vi "ARI Control.vi"(4 "Joystick Values":T2) -> (1 "Lifter Status":T1)   [LabVIEW 2014]
uses:
  <vilib>/Rock Robotics/WPI/Relay/WPI_RelayValue.ctl
panel:
  in  "Lifter Status Def":T1
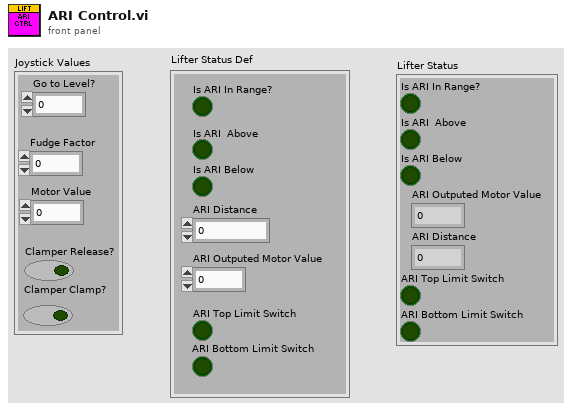
[diagram p1: front panel]
types:
  T1 = cluster{"Is ARI In Range?":bool, "Is ARI  Above":bool, "Is ARI Below":bool, "ARI Outputed Motor Value":dbl, "ARI Distance":dbl, "ARI Top Limit Switch":bool, "ARI Bottom Limit Switch":bool}
  T2 = cluster{"Go to Level?":i32, "Fudge Factor":dbl, "Clamper Release?":bool, "Motor Value":dbl, "Clamper Clamp?":bool}
  T3 = typedef "WPI_SwitchDevRef.ctl" = cluster{"DevStatus":errorcluster, "DIO Channel":T4, "Controller":T5, "CntIndex":T6, "Normally Closed":bool}
  T4 = typedef "FPGA_DIOChannel.ctl" = enum8{"DIO 0", "DIO 1", "DIO 2", "DIO 3", "DIO 4", "DIO 5", "DIO 6", "DIO 7", "DIO 8", "DIO 9", "DIO MXP 0", "DIO MXP 1", "DIO MXP 2", "DIO MXP 3", "DIO MXP 4", "DIO MXP 5", "DIO MXP 6", "DIO MXP 7", "DIO MXP 8", "DIO MXP 9", "DIO MXP 10", "DIO MXP 11", "DIO MXP 12", "DIO MXP 13", "DIO MXP 14", "DIO MXP 15", "Invalid"}
  T5 = typedef "FPGA_TypedefDigitalModule.ctl" = enum16{"Controller 1"}
  T6 = typedef "FPGA_CounterCtrSystemIndex.ctl" = enum8{"Ctr 0", "Ctr 1", "Ctr 2", "Ctr 3", "Ctr 4", "Ctr 5", "Ctr 6", "Ctr 7", "Invalid"}
  T7 = typedef "WPI_RelayValue.ctl" = enum16{"Off", "On", "Forward", "Reverse"}
  T8 = typedef "WPI_RelayDevRef.ctl" = cluster{"DevStatus":errorcluster, "Relay Channel":T9, "Controller":T5, "Relay Direction":T10}
  T9 = typedef "FPGA_DIORelayChannel.ctl" = enum8{"Relay 0", "Relay 1", "Relay 2", "Relay 3", "Invalid"}
  T10 = typedef "WPI_RelayDirection.ctl" = enum16{"Both directions", "Forward only", "Reverse only"}
  T11 = typedef "WPI_MotorControlDeviceRef.ctl" = cluster{"DeviceStatus":errorcluster, "Type":T12, "PWM":cluster{"Controller":T5, "PWM Channel":T13, "DeadBand":T14}, "CAN":cluster{"Device Number":u8, "Control Mode":T15, "Semaphore":T16, "Max Vout":dbl, "TalonSRX Control Mode":T17}, "Invert":bool, "TransformRef":T18, "InvTransformRef":T18}
  T12 = typedef "WPI_MotorControlType.ctl" = enum16{"PWM", "CAN", "CANTalonSRX"}
  T13 = typedef "FPGA_DIOPWMChannel.ctl" = enum8{"PWM 0", "PWM 1", "PWM 2", "PWM 3", "PWM 4", "PWM 5", "PWM 6", "PWM 7", "PWM 8", "PWM 9", "PWM MXP 0", "PWM MXP 1", "PWM MXP 2", "PWM MXP 3", "PWM MXP 4", "PWM MXP 5", "PWM MXP 6", "PWM MXP 7", "PWM MXP 8", "PWM MXP 9", "Invalid"}
  T14 = typedef "WPI_PWMDeadband.ctl" = cluster{"Name":string, "maxPositivePwm":i32, "minPositivePwm":i32, "centerPwm":i32, "maxNegativePwm":i32, "minNegativePwm":i32, "angularRange":u16}
  T15 = typedef "WPI_CANJaguar_ControlMode.ctl" = enum8{"Percent VBus", "Current", "Speed", "Position", "Voltage"}
  T16 = typedef "Semaphore RefNum" = refnum<k1>
  T17 = typedef "WPI_CANTalonSRX_APIControlMode.ctl" = enum8{"Percent VBus", "Speed", "Position", "Slave", "Unchanged / Invalid"}
  T18 = typedef "WPI_PWMTransform_ConPane.ctl" = refnum<vi>
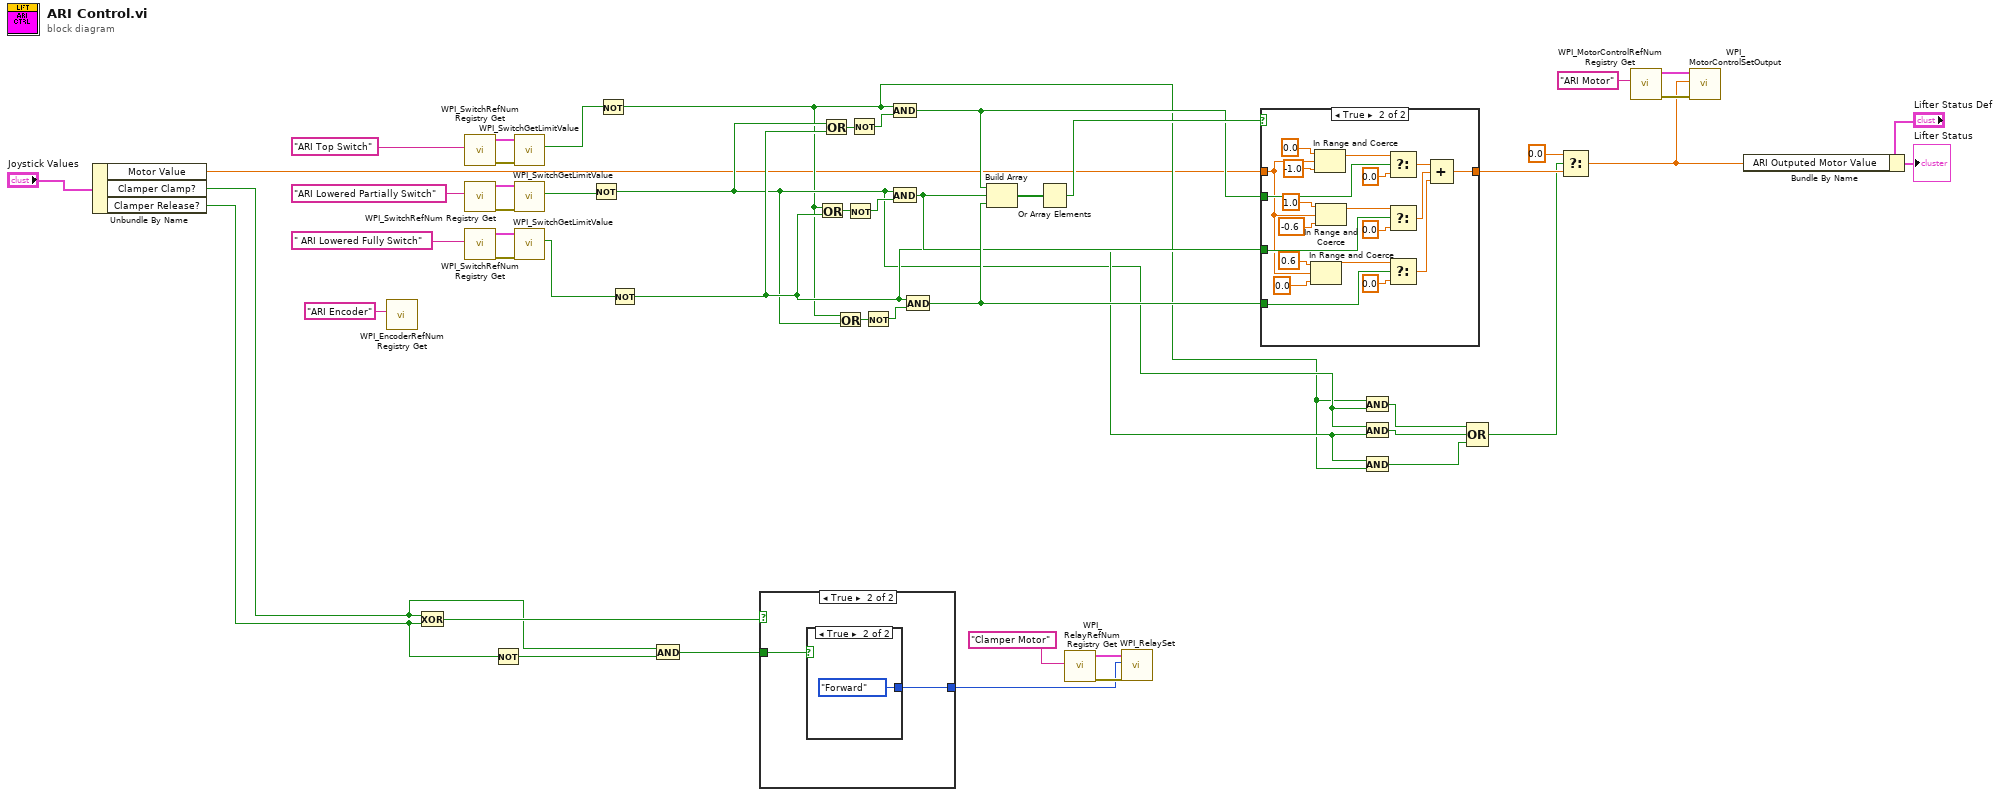
[diagram p0: block diagram]
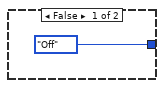
[diagram p3: hidden frame]
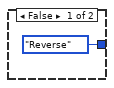
[diagram p4: hidden frame]
diagram:
  n1 = Unbundle By Name("Joystick Values") -> ("Motor Value"=w12:dbl, "Clamper Clamp?"=w2:bool, "Clamper Release?"=w4:bool)
  n2 = call <vilib>:"WPI_EncoderRefNum Registry Get.vi"("refnum name"="ARI Encoder") -> ()  [unwired: 9 in, 2 out]
  n3 = Exclusive Or(1:w4, 2:w2) -> (0:w6:bool)
  n4 = call <vilib>:"WPI_SwitchRefNum Registry Get.vi"("refnum name"="ARI Top Switch") -> ("error out"=w45:errorcluster, "SwitchDevRef"=w44:T3)  [unwired: 9 in]
  n5 = call <vilib>:"WPI_SwitchRefNum Registry Get.vi"("refnum name"="ARI Lowered Partially Switch") -> ("error out"=w42:errorcluster, "SwitchDevRef"=w43:T3)  [unwired: 9 in]
  n6 = call <vilib>:"WPI_SwitchRefNum Registry Get.vi"("refnum name"=" ARI Lowered Fully Switch") -> ("error out"=w38:errorcluster, "SwitchDevRef"=w37:T3)  [unwired: 9 in]
  n7 = Not(x=w4) -> (.not. x?=w3:bool)
  n8 = call <vilib>:"WPI_SwitchGetLimitValue.vi"("error in (no error)"=w45, "SwitchDevRef"=w44) -> ("Switch Pressed"=w9:bool)  [unwired: 7 in, 2 out]
  n9 = call <vilib>:"WPI_SwitchGetLimitValue.vi"("error in (no error)"=w42, "SwitchDevRef"=w43) -> ("Switch Pressed"=w10:bool)  [unwired: 7 in, 2 out]
  n10 = call <vilib>:"WPI_SwitchGetLimitValue.vi"("error in (no error)"=w38, "SwitchDevRef"=w37) -> ("Switch Pressed"=w11:bool)  [unwired: 7 in, 2 out]
  n11 = Not(x=w10) -> (.not. x?=w15:bool)
  n12 = Not(x=w9) -> (.not. x?=w14:bool)
  n13 = Not(x=w11) -> (.not. x?=w16:bool)
  n14 = And(x=w2, y=w3) -> (x .and. y?=w1:bool)
  n15 = case shown="True" w6 {
    tunnel: [WPI_RelayValue."Off" ("RelayValue") w52] -> w5
    tunnel: w1 -> [_ w53]
    frame False {
    }
    frame True {
      n16 = case shown="True" w53 {
        tunnel: [WPI_RelayValue."Reverse" ("RelayValue") WPI_RelayValue."Forward" ("RelayValue")] -> w52
        frame False {
        }
        frame True {
        }
      }
    }
  }
  n17 = Or(x=w14, y=w16) -> (x .or. y?=w31:bool)
  n18 = Or(x=w15, y=w16) -> (x .or. y?=w33:bool)
  n19 = Or(x=w14, y=w15) -> (x .or. y?=w29:bool)
  n20 = Not(x=w31) -> (.not. x?=w30:bool)
  n21 = Not(x=w33) -> (.not. x?=w32:bool)
  n22 = Not(x=w29) -> (.not. x?=w28:bool)
  n23 = And(x=w14, y=w32) -> (x .and. y?=w23:bool)
  n24 = And(x=w15, y=w30) -> (x .and. y?=w24:bool)
  n25 = And(x=w16, y=w28) -> (x .and. y?=w25:bool)
  n26 = Build Array(w23, w24, w25) -> (w27:bool[])
  n27 = Or Array Elements(Boolean array=w27) -> (logical OR=w26:bool)
  n28 = call <vilib>:"WPI_RelayRefNum Registry Get.vi"("refnum name"="Clamper Motor") -> ("error out"=w8:errorcluster, "RelayDevRef"=w7:T8)  [unwired: 9 in]
  n29 = call <vilib>:"WPI_RelaySet.vi"("error in (no error)"=w8, "RelayValue"=w5, "RelayDevRef"=w7) -> ()  [unwired: 7 in, 2 out]
  n30 = case shown="True" w26 {
    tunnel: [w56 w58] -> w22
    tunnel: w12 -> [w56 w57]
    tunnel: w25 -> [_ w76]
    tunnel: w23 -> [_ w75]
    tunnel: w24 -> [_ w74]
    frame False {
    }
    frame True {
      n31 = In Range and Coerce(upper limit=0.6, x=w57, lower limit=0.0) -> (coerced(x)=w69:dbl)  [unwired: 1 out]
      n32 = In Range and Coerce(upper limit=0.0, x=w57, lower limit=-1.0) -> (coerced(x)=w65:dbl)  [unwired: 1 out]
      n33 = In Range and Coerce(upper limit=1.0, x=w57, lower limit=-0.6) -> (coerced(x)=w71:dbl)  [unwired: 1 out]
      n34 = Select(t=w65, s=w75, f=0.0) -> (s? t:f=w61:dbl)
      n35 = Select(t=w71, s=w74, f=0.0) -> (s? t:f=w60:dbl)
      n36 = Select(t=w69, s=w76, f=0.0) -> (s? t:f=w59:dbl)
      n37 = Compound Arithmetic op=ADD(w61, w60, w59) -> (w58:dbl)
    }
  }
  n38 = And(x=w14, y=w15) -> (x .and. y?=w20:bool)
  n39 = And(x=w15, y=w16) -> (x .and. y?=w19:bool)
  n40 = And(x=w16, y=w14) -> (x .and. y?=w18:bool)
  n41 = Compound Arithmetic op=OR(w20, w19, w18) -> (w17:bool)
  n42 = Select(t=0.0, s=w17, f=w22) -> (s? t:f=w13:dbl)
  n43 = call <vilib>:"WPI_MotorControlRefNum Registry Get.vi"("refnum name"="ARI Motor") -> ("error out"=w34:errorcluster, "MotorControlDevRef"=w35:T11)  [unwired: 9 in]
  n44 = call <vilib>:"WPI_MotorControlSetOutput.vi"("error in (no error)"=w34, "Output"=w13, "MotorControlDevRef"=w35) -> ()  [unwired: 6 in, 3 out]
  n45 = Bundle By Name(cluster="Lifter Status Def", "ARI Outputed Motor Value"=w13) -> (→"Lifter Status":T1)
